vi "thermo_declusterize.vi"(0 "temp channel":T1[][](array[typedef])) -> (1 "temperature":dbl[][](array[numeric]), 2 "RH":dbl[][](array[numeric]), 3 "pressure":dbl[][](array[numeric]))   [LabVIEW 2020]
uses:
  thermo_read.ctl
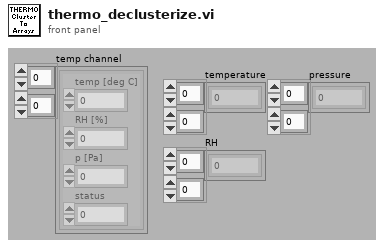
[diagram p1: front panel]
types:
  T1 = typedef "thermo_read.ctl" = cluster{"temp [deg C]":dbl, "RH [%]":dbl, "p [Pa]":dbl, "status":i32}
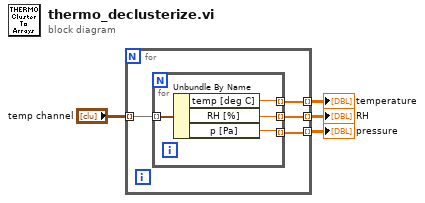
[diagram p0: block diagram]
diagram:
  n1 = for {
    tunnel: "temp channel" -> [w8] mode=indexing
    tunnel: [w7] -> w3 mode=indexing
    tunnel: [w6] -> w2 mode=indexing
    tunnel: [w5] -> w1 mode=indexing
    n2 = for {
      tunnel: w8 -> [w12] mode=indexing
      tunnel: [w11] -> w7 mode=indexing
      tunnel: [w10] -> w6 mode=indexing
      tunnel: [w9] -> w5 mode=indexing
      n3 = Unbundle By Name(w12) -> ("temp [deg C]"=w11:dbl, "RH [%]"=w10:dbl, "p [Pa]"=w9:dbl)
    }
  }
  "temperature" <- w3
  "RH" <- w2
  "pressure" <- w1
